vi "Open Base System Definition.vi"(8 "error in (no error)":errorcluster) -> (0 "error out":errorcluster, 2 "SLSC Custom Device  Ref out":T1 format="%.0x", 3 "SystemDefinition":refnum<k24>)   [LabVIEW 2017, in "SLSC Switch Scripting System Tests.lvclass"]
uses:
  SLSC Switch Scripting System Tests.lvclass
  <vilib>/NI Veristand/Custom Device API/Custom Device Item Ref.ctl
  NationalInstruments.VeriStand.SystemDefinitionAPI
  <userlib>/_OpenG.lib/file/file.llb/Append Path to Root if Relative - Scalar__ogtk.vi
  niveristand-custom-device-testing-tools/VeriStandTestUtilities/VeriStandTestUtilities.lvlib
  SLSC Switch Scripting.lvlib
  <vilib>/NI Veristand/Custom Device API/Custom Device API.lvlib
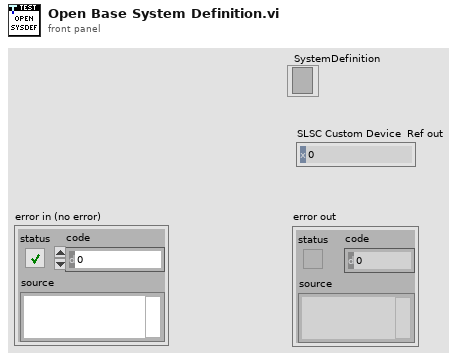
[diagram p1: front panel]
types:
  T1 = typedef "Custom Device API.lvlib/Custom Device Item Ref.ctl" = u64
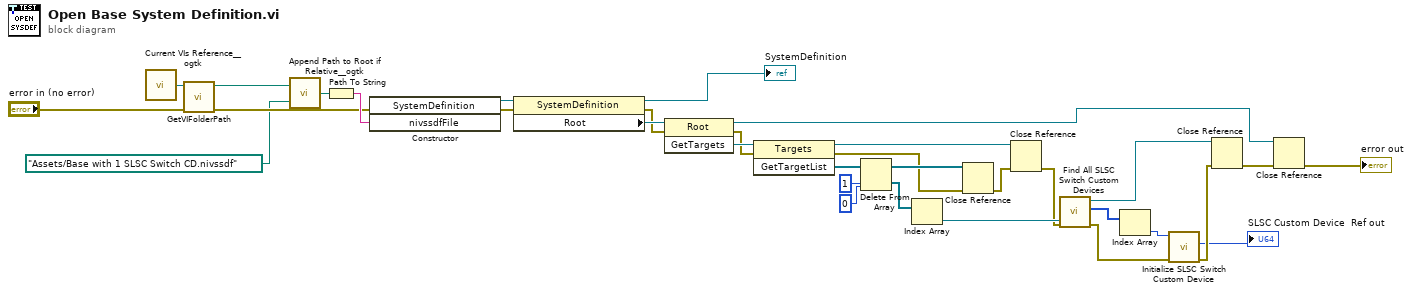
[diagram p0: block diagram]
diagram:
  n1 = call <userlib>:"Current VIs Reference__ogtk.vi"() -> ("Current VI's reference"=w13:refnum<vi>)  [unwired: 5 in]
  n2 = call "GetVIFolderPath.vi"("error in (no error)"="error in (no error)", "VI Reference in"=w13) -> ("error out"=w17:errorcluster, "VI Folder Path out"=w14:path)  [unwired: 8 in]
  n3 = call-poly <userlib>:"Append Path to Root if Relative__ogtk.vi"("Absolute or Relative Path"=path "Assets/Base with 1 SLSC Switch CD.nivssdf", "Root Path"=w14) -> ("Absolute or Appended Path"=w16:path)
  n4 = Path To String(path=w16) -> (string=w19:string)
  n5 = constructor class="SystemDefinition"(error in=w17, "nivssdfFile"=w19) -> (reference out=w20:refnum<k24>, error out=w18:errorcluster)  [unwired: 2 in, 2 out]
  n6 = property class="SystemDefinition"(reference=w20, error in=w18) -> (reference out=→"SystemDefinition":refnum<k24>, error out=w21:errorcluster, "Root"=w22:refnum<k24>)
  n7 = invoke class="Root" method="GetTargets"(reference=w22, error in=w21) -> (reference out=w9:refnum<k24>, error out=w23:errorcluster, "GetTargets"=w24:refnum<k24>)  [unwired: 1 in]
  n8 = invoke class="Targets" method="GetTargetList"(reference=w24, error in=w23) -> (reference out=w31:refnum<k24>, error out=w28:errorcluster, "GetTargetList"=w25:refnum<k24>[])  [unwired: 1 in]
  n9 = Delete From Array(array=w25, length=1, index=0) -> (deleted portion=w32:refnum<k24>[], array with subset deleted=w29:refnum<k24>[])
  n10 = Index Array(array=w32) -> (element=w8:refnum<k24>)  [unwired: 1 in]
  n11 = Close Reference(reference=w29, error in (no error)=w28) -> (error out=w30:errorcluster)
  n12 = Close Reference(reference=w31, error in (no error)=w30) -> (error out=w4:errorcluster)
  n13 = call "Find All SLSC Switch Custom Devices.vi"("error in (no error)"=w4, "Target in"=w8) -> ("error out"=w3:errorcluster, "SLSC Switch Custom Device Ref IDs"=w6:T1[], "Target out"=w7:refnum<k24>)  [unwired: 7 in]
  n14 = Index Array(array=w6) -> (element=w5:T1)  [unwired: 1 in]
  n15 = call "Initialize SLSC Switch Custom Device.vi"("error in (no error)"=w3, "SLSC Custom Device Ref in"=w5) -> ("error out"=w2:errorcluster, "Endpoint Configuration Section Ref"=→"SLSC Custom Device  Ref out":T1)  [unwired: 7 in, 1 out]
  n16 = Close Reference(reference=w7, error in (no error)=w2) -> (error out=w11:errorcluster)
  n17 = Close Reference(reference=w9, error in (no error)=w11) -> (error out=→"error out":errorcluster)
